vi "MyOwnStartStopIntegration.vi"(8 "Error In":errorcluster, 10 "Start/Stop":bool, 11 "VISA resource name":refnum<visa-resource-name>) -> (0 "Error Out":errorcluster, 3 "VISA resource name 2":refnum<visa-resource-name>)   [LabVIEW 2013, in "Universal Power Meter.lvlib" / "Yokogawa WT2X0.lvlib" / "Yokogawa WT2X0.lvclass"]
uses:
  Yokogawa WT2X0.lvclass
  <instrlib>/Yokogawa WT200 Series/Yokogawa WT200 Series.lvlib
panel:
  out "output string":string
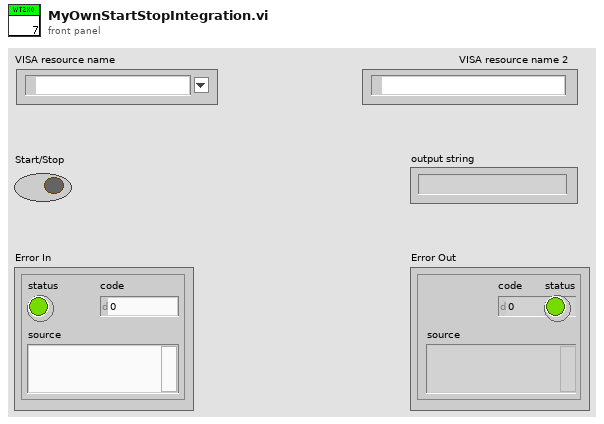
[diagram p1: front panel]
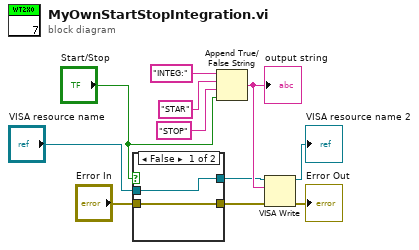
[diagram p0: block diagram]
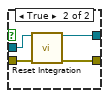
[diagram p2: hidden frame]
diagram:
  n1 = case shown="False" "Start/Stop" {
    tunnel: [w12 w17] -> w4
    tunnel: [w13 w16] -> w3
    tunnel: "VISA resource name" -> [w13 w15]
    tunnel: "Error In" -> [w12 w14]
    frame False {
    }
    frame True {
      n2 = call <instrlib>:"Reset Integration.vi"("VISA resource name"=w15, "error in (no error)"=w14) -> ("VISA resource name out"=w16:refnum<visa-resource-name>, "error out"=w17:errorcluster)  [unwired: 12 in]
    }
  }
  n3 = Append True/False String(1:"Start/Stop", 2:"STOP", 3:"STAR", 4:"INTEG:") -> (0:w9:string)
  "output string" <- w9
  n4 = VISA Write(VISA resource name=w3, write buffer=w9, error in (no error)=w4) -> (VISA resource name out=→"VISA resource name 2":refnum<visa-resource-name>, error out=→"Error Out":errorcluster)  [unwired: 1 out]
